vi "Execute.vi"(0 "SegmentSequencer in":refnum<class "SegmentSequencer.lvclass">, 3 "start":bool, 4 "reset":bool, 6 "continuous?":bool, 7 "req fifo":i16) -> (10 "state":T1, 14 "SegmentSequencer out":refnum<class "SegmentSequencer.lvclass">, 16 "step counter":u32, 17 "repeat counter":u64, 18 "Loaded steps":u32, 19 "generated requests":i64)   [LabVIEW 2019, in "TX burst sequencer.lvlib" / "SegmentSequencer.lvclass"]
uses:
  SegmentSequencer.lvclass
  FPGA sequencer states.ctl
  SegmentSequencer.lvclass/SegmentSequencer.ctl
  FPGA sequencer loopdata.ctl
  FPGA sequence step.ctl
  <vilib>/rvi/DataTransferAndStorage/Container/Common/niFpgaContainerExecOnDevCompGetState.vi
  <vilib>/rvi/Emulation/niFpgaEmulationIsFPGAContextNoSignature.vi
  <vilib>/rvi/DataTransferAndStorage/Container/Common/niFpgaContainerGetUniqueNameForEmu.vi
  <vilib>/rvi/Memory/Memory_Emulation/niFpgaMemoryEmulationCacheClearOnFirstRun.vi
  <vilib>/rvi/Memory/Memory_Emulation/nirvimemoryEmulationManagerCache_MakeExclusive.vi
  <vilib>/rvi/Memory/Memory_Emulation/niFpgaMemoryEmulationValidateCache.vi
  <vilib>/rvi/Memory/Memory_Emulation/nirvimemoryEmulationManagerCache_InsertValue.vi
  <vilib>/Utility/error.llb/Clear Errors.vi
  <vilib>/rvi/Memory/Memory_Emulation/nirvimemoryEmulationManagerCache_ReleaseExclusive.vi
  <vilib>/rvi/Memory/Memory_Emulation/nirvimemoryEmulationManagerCache_GetValue.vi
  <vilib>/rvi/Memory/Memory_Emulation/nirvimemoryEmulationManagerCache_SetValue.vi
  <vilib>/rvi/Emulation/niFpgaProcessEmulError.vi
  <vilib>/rvi/Emulation/niFpgaSctlEmulationGetInTimedLoop.vi
  <vilib>/rvi/errors/nirviReportUnexpectedCaseInternalError (U32).vi
  <vilib>/rvi/Emulation/niFpgaSctlEmulationResourceMgr.vi
  <vilib>/rvi/errors/niFpgaSetErrorForExecOnDevCompSimple.vi
  <vilib>/rvi/eio/common/nirviEmuReportErrorAndStop.vi
  <vilib>/rvi/FIFO/Fifo_Resource/nirvififoEmulationSetSize.vi
  <vilib>/rvi/FIFO/Fifo_Resource/nirviFifoEmulationQueueMgr.vi
  <instcachedir>/0/nirviFifoEmulationQueueMgr_E5CAEC123FF24DC58D834DCA3CDAA9B5.lvgen/nirviFifoEmulationQueueMgr_E5CAEC123FF24DC58D834DCA3CDAA9B5_003.vi
  <vilib>/rvi/FIFO/Fifo_Resource/nirvififoEmulationDetermineInputValidOut.vi
  <vilib>/rvi/FIFO/Fifo_Resource/nirvififoEmulationCreateLock.vi
  <vilib>/rvi/FIFO/Fifo_Resource/nirvififoEmulationObtainLock.vi
  <vilib>/rvi/FIFO/Fifo_Resource/nirvififoEmulationReleaseLock.vi
  <vilib>/rvi/occurrence/nirviWaitOnOccurrenceBase.vi
  <vilib>/rvi/errors/nirviReportUnexpectedCaseInternalError.vi
  <vilib>/rvi/interface/RandomDataEmulation/niFpgaRandomDataHandleErrors.vi
  <vilib>/rvi/DataTransferAndStorage/Container/XNode/niFpgaContainer.xnode
  <vilib>/rvi/DataTransferAndStorage/Register/Emulation/niFpgaRegisterEmulationRefIn.vi
  <vilib>/rvi/Memory/Memory_Emulation/niFpgaMemoryEmulationRefIn.vi
  <vilib>/rvi/FIFO/Fifo_Resource/niFpgaFifoEmulationRefIn.vi
  <instrlib>/_niInstr/Basic Elements/v1/FPGA/niInstr Basic Elements v1 FPGA.lvlib
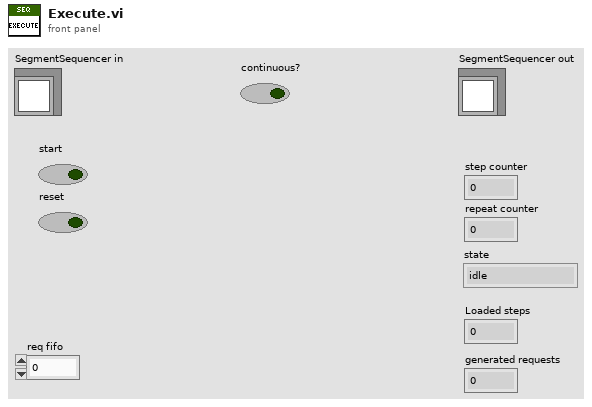
[diagram p1: front panel]
types:
  T1 = typedef "FPGA sequencer states.ctl" = enum16{"idle", "read step", "execute step"}
  T2 = typedef "TX burst sequencer.lvlib/SegmentSequencer.lvclass/FPGA sequencer loopdata.ctl" = cluster{"step counter":u32, "repeat counter":u64, "read ptr":u32, "active step":T3, "read cycles ctr":u8}
  T3 = typedef "TX burst sequencer.lvlib/SegmentSequencer.lvclass/FPGA sequence step.ctl" = cluster{"start addr":u32, "end addr":u32, "repeat":u64}
  T4 = cluster{"start addr":u32, "end addr":u32, "repeat":u64}
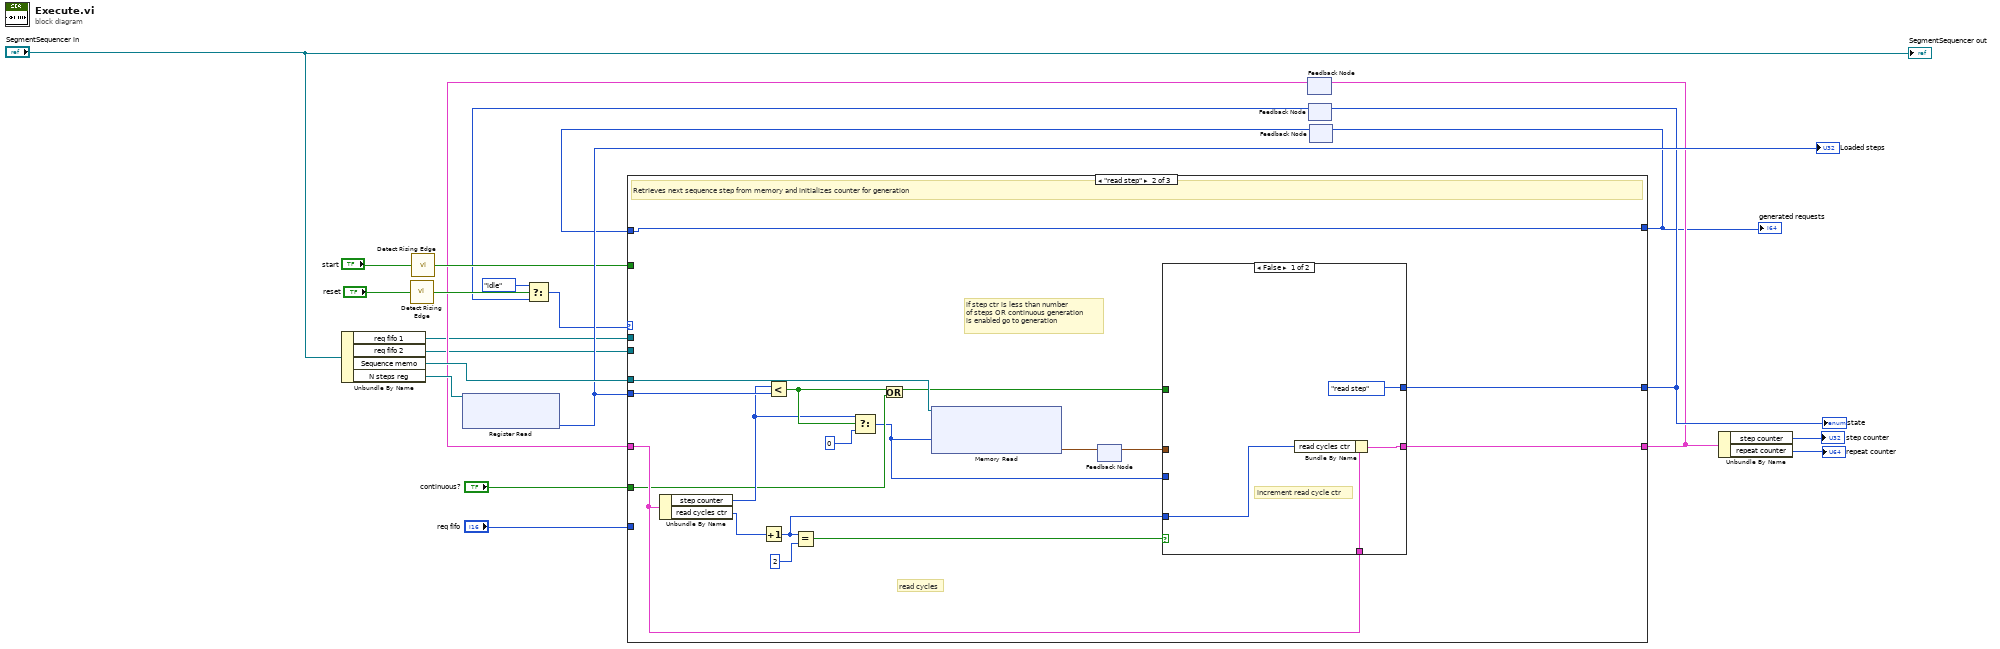
[diagram p0: block diagram]
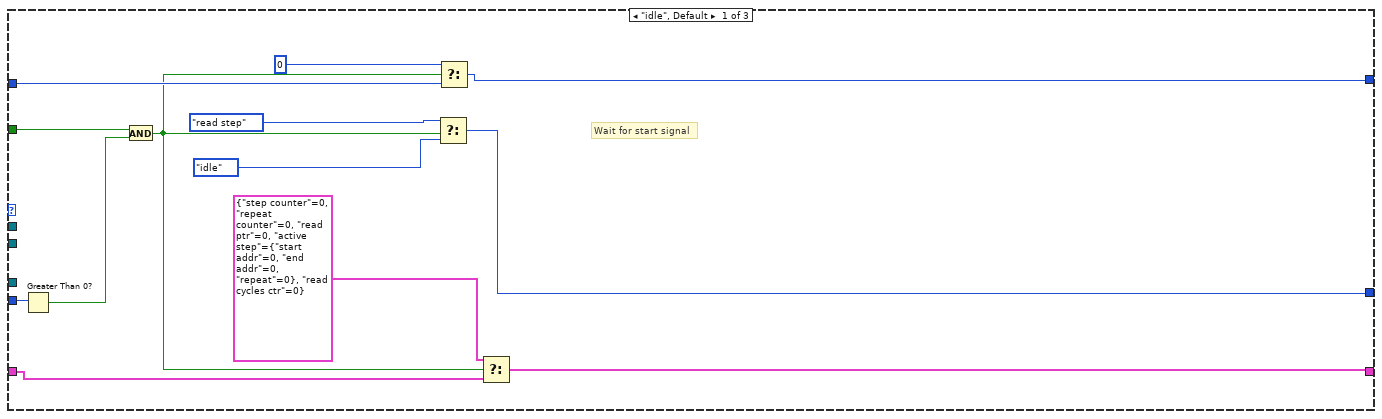
[diagram p2: hidden frame]
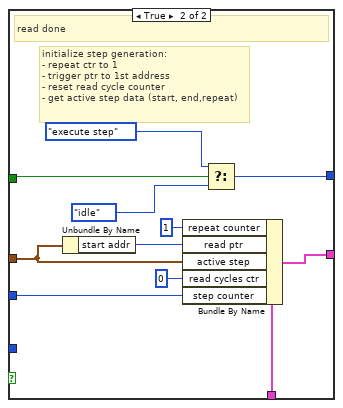
[diagram p3: hidden frame]
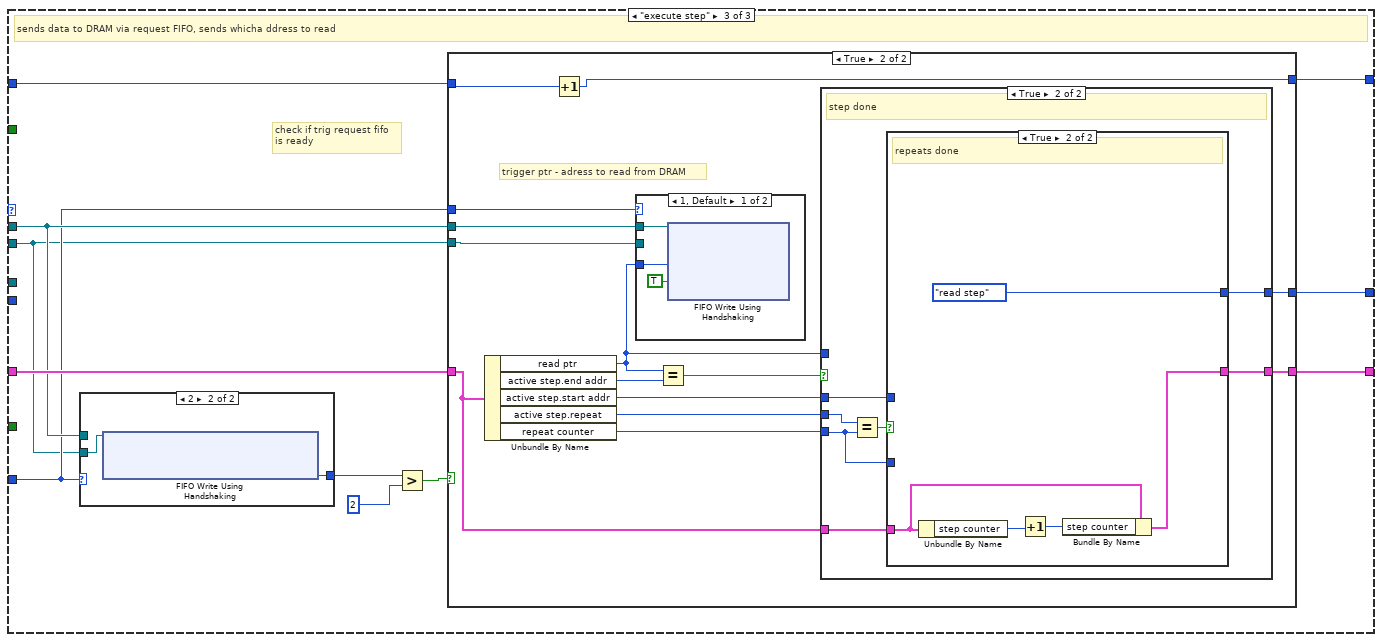
[diagram p4: hidden frame]
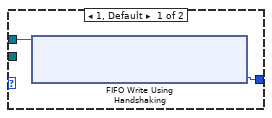
[diagram p5: hidden frame]
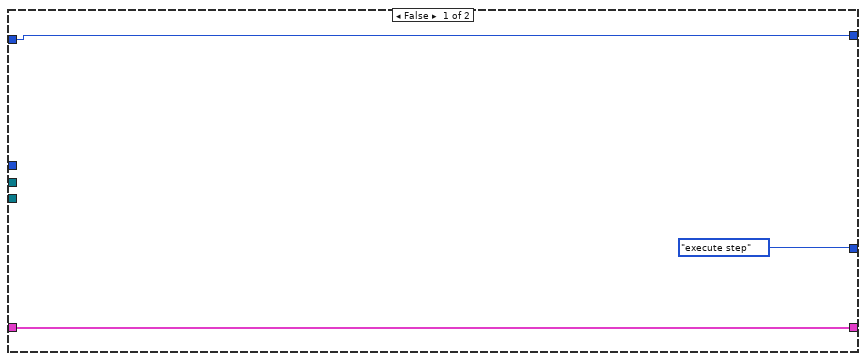
[diagram p6: hidden frame]
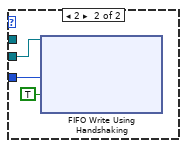
[diagram p7: hidden frame]
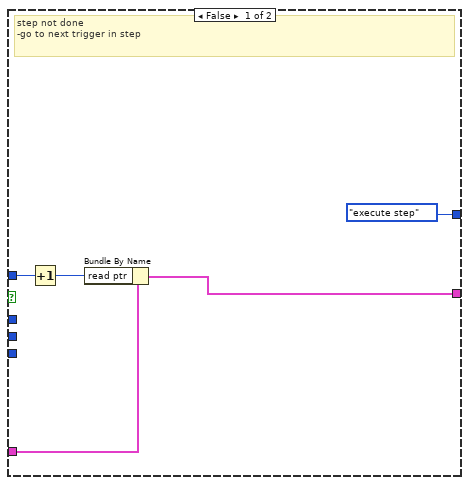
[diagram p8: hidden frame]
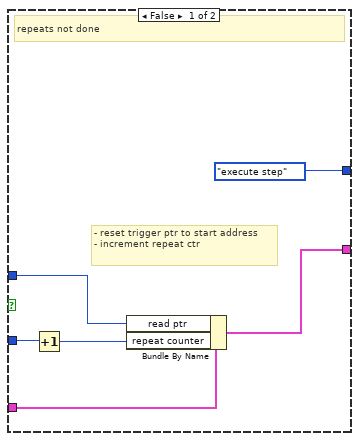
[diagram p9: hidden frame]
diagram:
  n1 = Unbundle By Name("SegmentSequencer in") -> ("req fifo 1"=w6:refnum<k21>, "req fifo 2"=w2:refnum<k21>, "Sequence memo"=w22:refnum<k21>, "N steps reg"=w21:refnum<k21>)
  n2 = call <instrlib>:"Detect Rising Edge.vi"("signal"="reset") -> ("edge detected"=w14:bool)  [unwired: 14 in]
  n3 = call <instrlib>:"Detect Rising Edge.vi"("signal"="start") -> ("edge detected"=w15:bool)  [unwired: 14 in]
  n4 = xnode ("Register Read")("Register In"=w21) -> ("Data"=w20:u32)  [unwired: 1 out]
  "Loaded steps" <- w20
  n5 = feedback #1() -> (w8:T2)  [unwired: 1 in]
  n6 = feedback #2() -> (w10:T1)  [unwired: 1 in]
  n7 = Select(t=FPGA_sequencer_states."idle", s=w14, f=w10) -> (s? t:f=w12:T1)
  n8 = feedback #3() -> (w4:i64)  [unwired: 1 in]
  n9 = case shown="\"read step\"" w12 {
    tunnel: [w33 w44 w76] -> w11
    tunnel: [w23 w47 w77] -> w9
    tunnel: w8 -> [w26 w49 w78]
    tunnel: w22 -> [_ w53 _]
    tunnel: w6 -> [_ _ w71]
    tunnel: w20 -> [w32 w43 _]
    tunnel: w15 -> [w30 _ _]
    tunnel: [w27 w42 w72] -> w5
    tunnel: w4 -> [w29 w42 w73]
    tunnel: "continuous?" -> [_ w37 _]
    tunnel: w2 -> [_ _ w69]
    tunnel: "req fifo" -> [_ _ w70]
    frame "idle", Default {
      # "Wait for start signal"
      n10 = Greater Than 0?(x=w32) -> (x > 0?=w31:bool)
      n11 = And(x=w30, y=w31) -> (x .and. y?=w24:bool)
      n12 = Select(t=FPGA_sequencer_states."read step", s=w24, f=FPGA_sequencer_states."idle" ("t")) -> (s? t:f=w33:T1)
      n13 = Select(t=i64 0, s=w24, f=w29) -> (s? t:f=w27:i64)
      n14 = Select(t=T2 {"step counter"=0, "repeat counter"=0, "read ptr"=0, "active step"={"start addr"=0, "end addr"=0, "repeat"=0}, "read cycles ctr"=0} ("Sequencer data"), s=w24, f=w26) -> (s? t:f=w23:T2)
    }
    frame "read step" {
      # "if step ctr is less than number\nof steps OR continuous generation\nis enabled go to generation"
      # "read cycles"
      # "Retrieves next sequence step from memory and initializes counter for generation"
      n15 = Unbundle By Name(w49) -> ("step counter"=w38:u32, "read cycles ctr"=w52:u8)
      n16 = Increment(x=w52) -> (x+1=w45:u8)
      n17 = Less?(x=w38, y=w43) -> (x < y?=w40:bool)
      n18 = Equal?(x=w45, y=u8 2 ("x")) -> (x = y?=w48:bool)
      n19 = Select(t=w38, s=w40, f=u32 0 ("t")) -> (s? t:f=w36:u32)
      n20 = Or(x=w40, y=w37) -> (x .or. y?=w41:bool)
      n21 = xnode ("Memory Read")("Address"=w36, "Memory In"=w53) -> ("Data"=w51:T4)  [unwired: 1 out]
      n22 = feedback-in #4(w51) -> ()
      n23 = feedback #4() -> (w46:T4)  [unwired: 1 in]
      n24 = case shown="False" w48 {
        tunnel: w49 -> [w57 w68]
        tunnel: [w55 w67] -> w47
        tunnel: w46 -> [_ w65]
        tunnel: w45 -> [w56 _]
        tunnel: [FPGA_sequencer_states."read step" w59] -> w44
        tunnel: w41 -> [_ w62]
        tunnel: w36 -> [_ w58]
        frame False {
          # "increment read cycle ctr"
          n25 = Bundle By Name(cluster=w57, "read cycles ctr"=w56) -> (w55:T2)
        }
        frame True {
          # "initialize step generation:\n- repeat ctr to 1\n- trigger ptr to 1st address\n- reset read cycle counter\n- get active step data (start, end,repeat)"
          # "read done"
          n26 = Unbundle By Name(w65) -> ("start addr"=w64:u32)
          n27 = Bundle By Name(cluster=w68, "repeat counter"=u64 1, "read ptr"=w64, "active step"=w65, "read cycles ctr"=u8 0, "step counter"=w58) -> (w67:T2)
          n28 = Select(t=FPGA_sequencer_states."execute step", s=w62, f=FPGA_sequencer_states."idle") -> (s? t:f=w59:T1)
        }
      }
    }
    frame "execute step" {
      # "check if trig request fifo\nis ready"
      # "sends data to DRAM via request FIFO, sends whicha ddress to read"
      n29 = case shown="2" w70 {
        tunnel: w71 -> [w81 _]
        tunnel: [w80 w82] -> w75
        tunnel: w69 -> [_ w83]
        frame 1, Default {
          n30 = xnode ("FIFO Write Using Handshaking")("FIFO In"=w81) -> ("Number of Elements to Write"=w80:u32)  [unwired: 1 out]
        }
        frame 2 {
          n31 = xnode ("FIFO Write Using Handshaking")("FIFO In"=w83) -> ("Number of Elements to Write"=w82:u32)  [unwired: 1 out]
        }
      }
      n32 = Greater?(x=w75, y=u32 2) -> (0:w79:bool)
      n33 = case shown="True" w79 {
        tunnel: w78 -> [w85 w96]
        tunnel: [w85 w95] -> w77
        tunnel: [FPGA_sequencer_states."execute step" w92] -> w76
        tunnel: w73 -> [w84 w91]
        tunnel: [w84 w90] -> w72
        tunnel: w71 -> [_ w89]
        tunnel: w70 -> [_ w88]
        tunnel: w69 -> [_ w87]
        frame False {
        }
        frame True {
          # "trigger ptr - adress to read from DRAM"
          n34 = Unbundle By Name(w96) -> ("read ptr"=w97:u32, "active step.end addr"=w100:u32, "active step.start addr"=w98:u32, "active step.repeat"=w94:u64, "repeat counter"=w93:u64)
          n35 = Increment(x=w91) -> (x+1=w90:i64)
          n36 = case shown="1, Default" w88 {
            tunnel: w97 -> [w102 w105]
            tunnel: w89 -> [w101 _]
            tunnel: w87 -> [_ w104]
            frame 1, Default {
              n37 = xnode ("FIFO Write Using Handshaking")("Element"=w102, "Input Valid"=TRUE, "FIFO In"=w101) -> ()  [unwired: 2 out]
            }
            frame 2 {
              n38 = xnode ("FIFO Write Using Handshaking")("Element"=w105, "Input Valid"=TRUE, "FIFO In"=w104) -> ()  [unwired: 2 out]
            }
          }
          n39 = Equal?(x=w97, y=w100) -> (x = y?=w99:bool)
          n40 = case shown="True" w99 {
            tunnel: w98 -> [_ w112]
            tunnel: w97 -> [w111 _]
            tunnel: w96 -> [w110 w115]
            tunnel: [w108 w114] -> w95
            tunnel: w94 -> [_ w118]
            tunnel: w93 -> [_ w113]
            tunnel: [FPGA_sequencer_states."execute step" w116] -> w92
            frame False {
              # "step not done\n-go to next trigger in step"
              n41 = Increment(x=w111) -> (x+1=w109:u32)
              n42 = Bundle By Name(cluster=w110, "read ptr"=w109) -> (w108:T2)
            }
            frame True {
              # "step done"
              n43 = Equal?(x=w118, y=w113) -> (x = y?=w117:bool)
              n44 = case shown="True" w117 {
                tunnel: [FPGA_sequencer_states."execute step" FPGA_sequencer_states."read step"] -> w116
                tunnel: w115 -> [w122 w127]
                tunnel: [w121 w125] -> w114
                tunnel: w113 -> [w124 _]
                tunnel: w112 -> [w119 _]
                frame False {
                  # "- reset trigger ptr to start address\n- increment repeat ctr"
                  # "repeats not done"
                  n45 = Increment(x=w124) -> (x+1=w120:u64)
                  n46 = Bundle By Name(cluster=w122, "read ptr"=w119, "repeat counter"=w120) -> (w121:T2)
                }
                frame True {
                  # "repeats done"
                  n47 = Unbundle By Name(w127) -> ("step counter"=w128:u32)
                  n48 = Increment(x=w128) -> (x+1=w126:u32)
                  n49 = Bundle By Name(cluster=w127, "step counter"=w126) -> (w125:T2)
                }
              }
            }
          }
        }
      }
    }
  }
  "state" <- w11
  "generated requests" <- w5
  n50 = feedback-in #1(w9) -> ()
  n51 = feedback-in #2(w11) -> ()
  n52 = feedback-in #3(w5) -> ()
  n53 = Unbundle By Name(w9) -> ("step counter"=→"step counter":u32, "repeat counter"=→"repeat counter":u64)
  "SegmentSequencer out" <- "SegmentSequencer in"
